vi "Baud.vi"(8 "error in":errorcluster, 9 "Baud Rate (BPS)":T2=enum."57600", 11 "UART port in":T1) -> (0 "error out":errorcluster, 3 "UART port out":T1)   [LabVIEW 2015]
doc: "Set the iRobot baud rate; the serial port will be reconfigured to this new baud rate and restarted, which will clear communication buffers and may introduce a delay.\n\nNote: Baud 115200 appears to be unstable.\n\nThis VI writes to, but does not read from, the serial port."
uses:
  Baud.ctl
  UART/iRobot UART Port Type.ctl
  OpCode.ctl
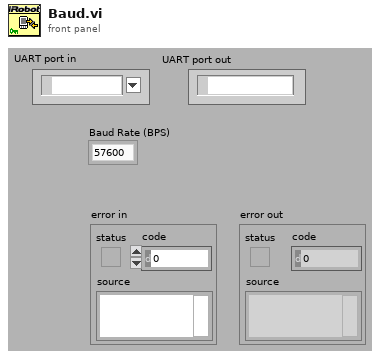
[diagram p1: front panel]
types:
  T1 = typedef "iRobot UART Port Type.ctl" = refnum<visa-resource-name>
  T2 = typedef "Baud.ctl" = enum8{"300", "600", "1200", "2400", "4800", "9600", "14400", "19200", "28800", "38400", "57600", "115200"}
  T3 = typedef "OpCode.ctl" = u8
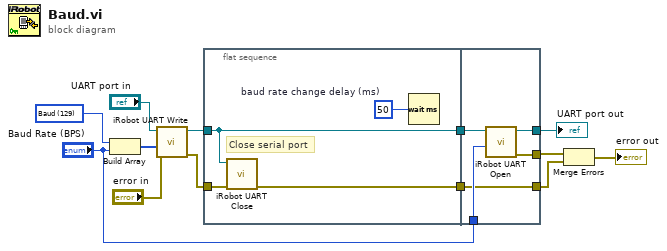
[diagram p0: block diagram]
diagram:
  w9 = T3 129 items=["Start"=128, "Baud"=129, "Control"=130, "Safe"=131, "Full"=132, "Demo"=136, "Demo - Cover"=135, "Demo - Cover and Dock"=143, "Demo - Spot"=134, "Drive"=137, "Drive Direct"=145, "LEDs"=139, "Digital Outputs"=147, "PWM Low Side Drivers"=144, "Low Side Drivers"=138, "Send IR"=151, "Song"=140, "Play Song"=141, "Sensors"=142, "Query List"=149, "Stream"=148, "Pause/Resume Stream"=150, "Script"=152, "Play Script"=153, "Show Script"=154, "Wait Time"=155, "Wait Distance"=156, "Wait Angle"=157, "Wait Event"=158] ("OpCode")
  n1 = Build Array(w9, "Baud Rate (BPS)") -> (w13:T3[])
  n2 = call "iRobot UART Write.vi"("error in"="error in", "data"=w13, "UART port in"="UART port in") -> ("error out"=w5:errorcluster, "UART port out"=w11:T1)  [unwired: 1 in, 6 out]
  n3 = flat-sequence {
    tunnel: w11 -> [w16]
    tunnel: [w16] -> w10
    tunnel: w5 -> [w15]
    tunnel: [w14] -> w4
    tunnel: w10 -> [w22]
    tunnel: [w21] -> w8
    tunnel: "Baud Rate (BPS)" -> [w20]
    tunnel: [w19] -> w3
    tunnel: [w18] -> w2
    tunnel: w4 -> [w18]
    frame #0 {
      w17 = u32 50  # baud rate change delay (ms)
      # "Close serial port"
      n4 = call "iRobot UART Close.vi"("error in"=w15, "UART port in"=w16) -> ("error out"=w14:errorcluster)  [unwired: 9 out]
      n5 = Wait (ms)(milliseconds to wait=w17) -> ()  [unwired: 1 out]
    }
    frame #1 {
      n6 = call "iRobot UART Open.vi"("Baud Rate (BPS)"=w20, "UART port in"=w22) -> ("error out"=w19:errorcluster, "UART port out"=w21:T1)  [unwired: 1 in, 7 out]
    }
  }
  n7 = Merge Errors(w3, w2) -> (→"error out":errorcluster)
  "UART port out" <- w8
